vi "Application Analyzer.vi"() -> ()   [LabVIEW 2019]
doc: "Analyzes progress and status of application."
uses:
  <vilib>/Utility/error.llb/DialogType.ctl
  <vilib>/Utility/miscctls.llb/LVPointTypeDef.ctl
panel:
  out "Control Tab":T1(tab)
  out "Files & Revision":string[][](array[string])
  out "Total Revisions":u32
  out "Error Message":string
  out "Error Out":errorcluster
  out "VI-filename":string
  out "VI Path":path
  out "Revision Number":u32
  in  "Tool Bar:Visible":bool
  in  "Tabs Visible?":bool
  out "VI-Name":string
  # "Settings"
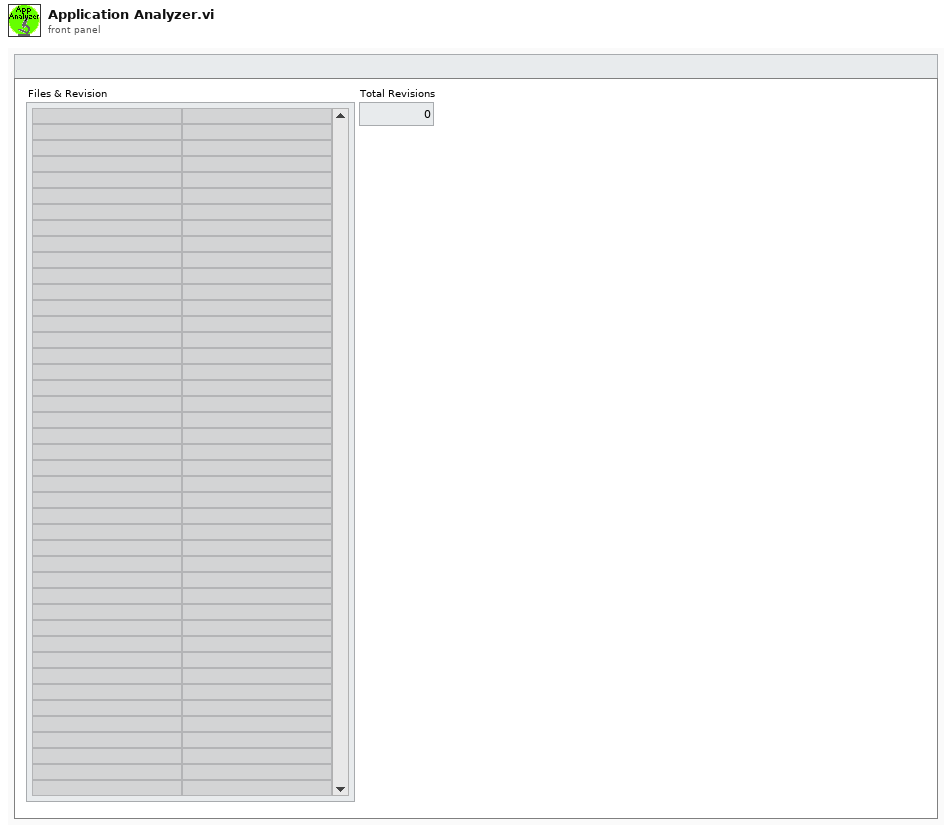
[diagram p1: front panel]
types:
  T1 = enum32{"GUI", "Controls & Indicators", "Error IO", "VI"}
  T2 = typedef "LVPointTypeDef.ctl" = cluster{"Horizontal":i16, "Vertical":i16}
  T3 = typedef "DialogType.ctl" = u16
  T4 = typedef "LVRectTypeDef.ctl" = cluster{"Left":i16, "Top":i16, "Right":i16, "Bottom":i16}
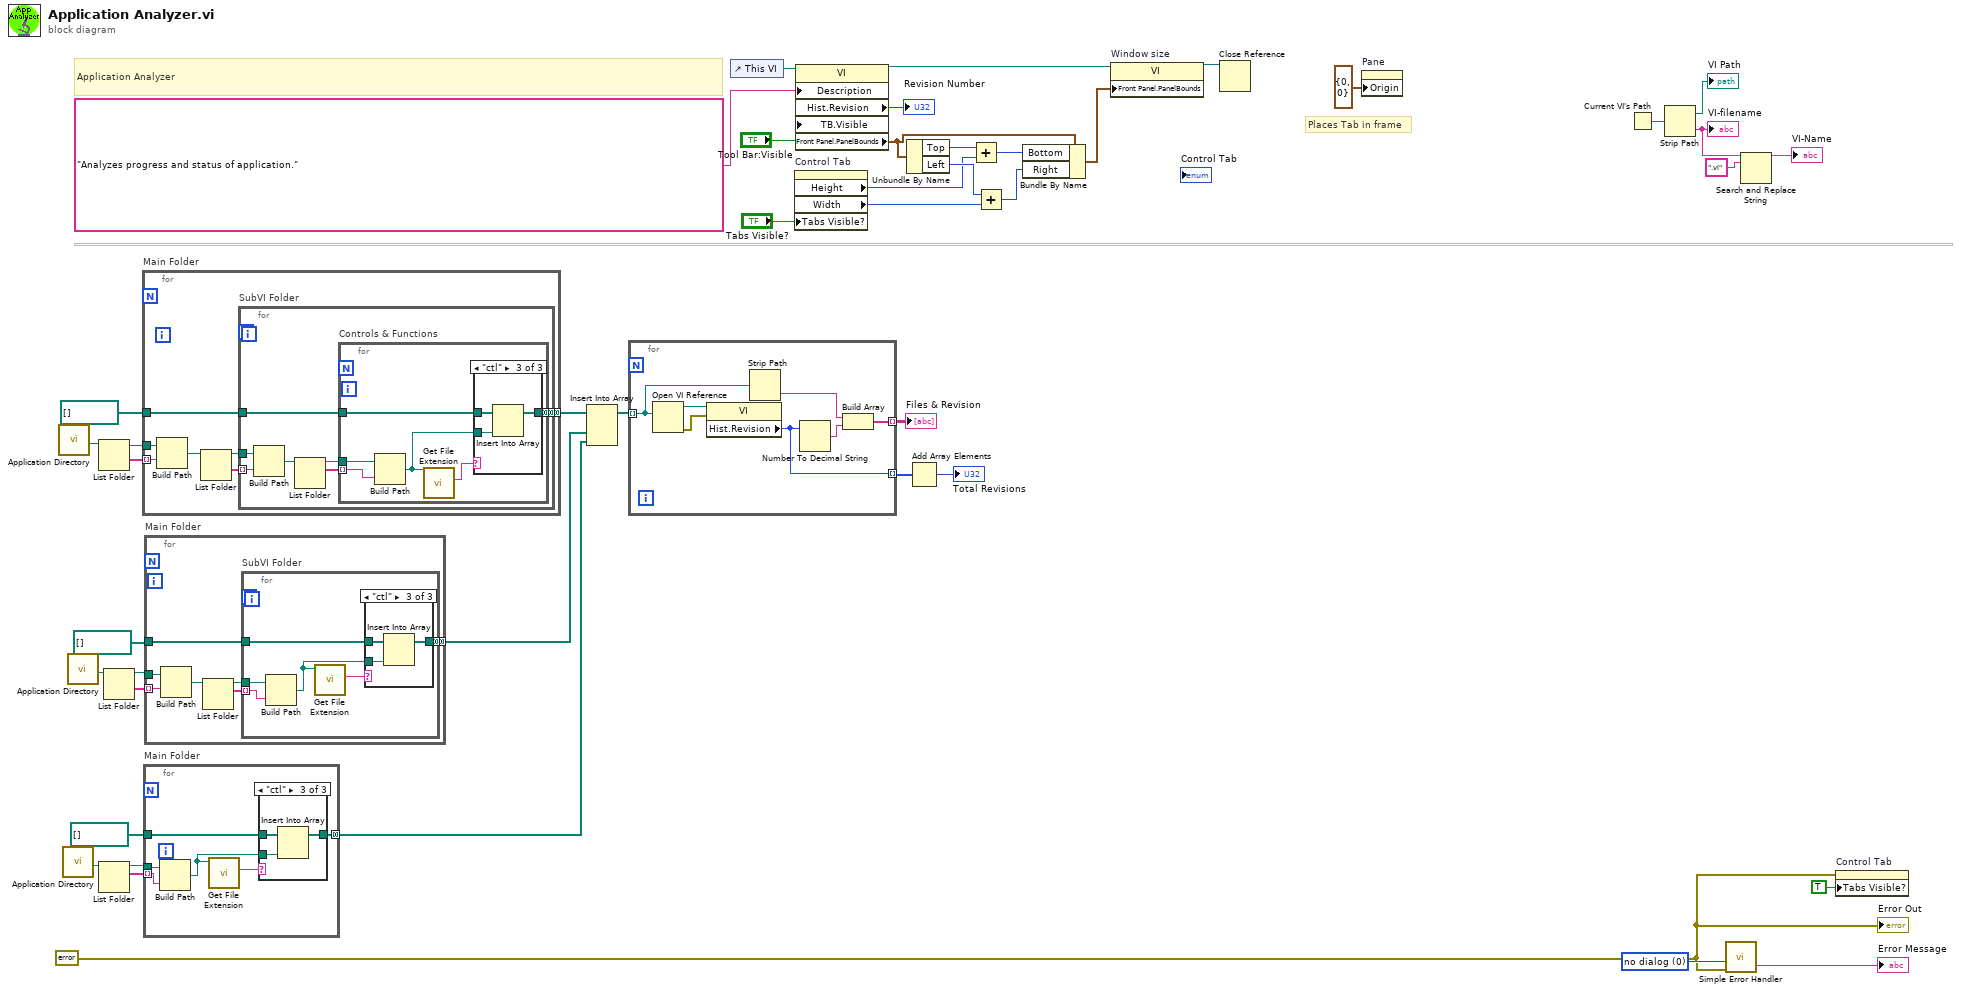
[diagram p0: block diagram]
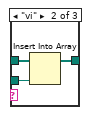
[diagram p3: hidden frame]
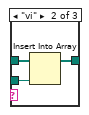
[diagram p5: hidden frame]
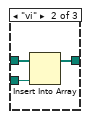
[diagram p7: hidden frame]
diagram:
  w32 = errorcluster {"status"=FALSE, "code"=0, "source"=""} ("Error In")
  w35 = T3 0 items=["no dialog", "OK message", "continue or stop message", "OK message + warnings", "continue/stop + warnings"] ("type of dialog (OK msg:1)")
  # "Places Tab in frame"
  # "Application Analyzer"
  n1 = call <vilib>:"Application Directory.vi"() -> ("Application Directory"=w17:path)
  n2 = call <vilib>:"Application Directory.vi"() -> ("Application Directory"=w12:path)
  n3 = call <vilib>:"Application Directory.vi"() -> ("Application Directory"=w16:path)
  n4 = List Folder(path=w17) -> (path out=w18:path, folder names=w19:string[])  [unwired: 3 in, 2 out]
  n5 = List Folder(path=w12) -> (path out=w13:path, filenames=w11:string[])  [unwired: 3 in, 2 out]
  n6 = List Folder(path=w16) -> (path out=w15:path, folder names=w14:string[])  [unwired: 3 in, 2 out]
  n7 = for "Main Folder" {
    tunnel: w19 -> [w51] mode=indexing
    tunnel: w18 -> [w46]
    tunnel: path[] [] -> [w47]
    tunnel: [w45] -> w6 mode=concatenating
    n8 = Build Path(base path=w46, name or relative path=w51) -> (appended path=w50:path)
    n9 = List Folder(path=w50) -> (path out=w48:path, folder names=w49:string[])  [unwired: 3 in, 2 out]
    n10 = for "SubVI Folder" {
      tunnel: w49 -> [w57] mode=indexing
      tunnel: w48 -> [w54]
      tunnel: w47 -> [w53]
      tunnel: [w52] -> w45 mode=concatenating
      n11 = Build Path(base path=w54, name or relative path=w57) -> (appended path=w58:path)
      n12 = List Folder(path=w58) -> (path out=w55:path, filenames=w56:string[])  [unwired: 3 in, 2 out]
      n13 = for "Controls & Functions" {
        tunnel: w56 -> [w62] mode=indexing
        tunnel: w55 -> [w64]
        tunnel: w53 -> [w61]
        tunnel: [w59] -> w52 mode=concatenating
        n14 = Build Path(base path=w64, name or relative path=w62) -> (appended path=w60:path)
        n15 = call <vilib>:"Get File Extension.vi"("file"=w60) -> ("lowercase file extension"=w63:string)  [unwired: 6 in, 4 out]
        n16 = case shown="\"ctl\"" w63 {
          tunnel: w61 -> [w65 w68 w71]
          tunnel: w60 -> [_ w66 w70]
          tunnel: [w65 w67 w69] -> w59
          frame "Other", Default {
          }
          frame "vi" {
            n17 = Insert Into Array(array=w68, new element=w66) -> (w67:path[])  [unwired: 1 in]
          }
          frame "ctl" {
            n18 = Insert Into Array(array=w71, new element=w70) -> (w69:path[])  [unwired: 1 in]
          }
        }
      }
    }
  }
  n19 = for "Main Folder" {
    tunnel: w13 -> [w73]
    tunnel: path[] [] -> [w77]
    tunnel: [w76] -> w4 mode=concatenating
    tunnel: w11 -> [w72] mode=indexing
    n20 = Build Path(base path=w73, name or relative path=w72) -> (appended path=w74:path)
    n21 = call <vilib>:"Get File Extension.vi"("file"=w74) -> ("lowercase file extension"=w75:string)  [unwired: 6 in, 4 out]
    n22 = case shown="\"ctl\"" w75 {
      tunnel: w77 -> [w78 w81 w84]
      tunnel: w74 -> [_ w79 w83]
      tunnel: [w78 w80 w82] -> w76
      frame "Other", Default {
      }
      frame "vi" {
        n23 = Insert Into Array(array=w81, new element=w79) -> (w80:path[])  [unwired: 1 in]
      }
      frame "ctl" {
        n24 = Insert Into Array(array=w84, new element=w83) -> (w82:path[])  [unwired: 1 in]
      }
    }
  }
  n25 = for "Main Folder" {
    tunnel: w14 -> [w91] mode=indexing
    tunnel: w15 -> [w86]
    tunnel: path[] [] -> [w87]
    tunnel: [w85] -> w5 mode=concatenating
    n26 = Build Path(base path=w86, name or relative path=w91) -> (appended path=w90:path)
    n27 = List Folder(path=w90) -> (path out=w89:path, filenames=w88:string[])  [unwired: 3 in, 2 out]
    n28 = for "SubVI Folder" {
      tunnel: w89 -> [w93]
      tunnel: w88 -> [w92] mode=indexing
      tunnel: w87 -> [w97]
      tunnel: [w96] -> w85 mode=concatenating
      n29 = Build Path(base path=w93, name or relative path=w92) -> (appended path=w94:path)
      n30 = call <vilib>:"Get File Extension.vi"("file"=w94) -> ("lowercase file extension"=w95:string)  [unwired: 6 in, 4 out]
      n31 = case shown="\"ctl\"" w95 {
        tunnel: w97 -> [w98 w101 w104]
        tunnel: w94 -> [_ w99 w103]
        tunnel: [w98 w100 w102] -> w96
        frame "Other", Default {
        }
        frame "vi" {
          n32 = Insert Into Array(array=w101, new element=w99) -> (w100:path[])  [unwired: 1 in]
        }
        frame "ctl" {
          n33 = Insert Into Array(array=w104, new element=w103) -> (w102:path[])  [unwired: 1 in]
        }
      }
    }
  }
  n34 = Insert Into Array(array=w6, new element #1=w5, new element #2=w4) -> (w3:path[])  [unwired: 1 in]
  n35 = for {
    tunnel: w3 -> [w111] mode=indexing
    tunnel: [w106] -> w2 mode=indexing
    tunnel: [w105] -> w10 mode=indexing
    n36 = Open VI Reference(vi path=w111) -> (vi reference=w109:refnum<vi>, error out=w110:errorcluster)  [unwired: 5 in]
    n37 = property class="VI"(reference=w109, error in=w110) -> ("Hist.Revision"=w106:u32)  [unwired: 2 out]
    n38 = Strip Path(path=w111) -> (name=w108:string)  [unwired: 1 out]
    n39 = Number To Decimal String(number=w106) -> (decimal integer string=w107:string)  [unwired: 1 in]
    n40 = Build Array(w108, w107) -> (w105:string[])
  }
  "Files & Revision" <- w10
  n41 = control-ref of="This VI"() -> (w41:refnum<vi>)
  n42 = property on="Control Tab" class="TabCtl (strict)"("Tabs Visible?"="Tabs Visible?") -> ("Height"=w26:u32, "Width"=w30:u32)  [unwired: 2 in, 2 out]
  n43 = property class="VI"(reference=w41, "Description"="Analyzes progress and status of application.", "TB.Visible"="Tool Bar:Visible") -> (reference out=w23:refnum<vi>, "Hist.Revision"=→"Revision Number":u32, "Front Panel.PanelBounds"=w24:T4)  [unwired: 1 in, 1 out]
  n44 = Unbundle By Name(w24) -> ("Top"=w25:i16, "Left"=w29:i16)
  n45 = Add Array Elements(numeric array=w2) -> (sum=→"Total Revisions":u32)
  n46 = Add(x=w25, y=w26) -> (x+y=w27:u32)
  n47 = Add(x=w29, y=w30) -> (x+y=w28:u32)
  n48 = Bundle By Name(cluster=w24, "Bottom"=w27, "Right"=w28) -> (w22:T4)
  n49 = property on="Window size" class="VI"(reference=w23, "Front Panel.PanelBounds"=w22) -> (reference out=w31:refnum<vi>)  [unwired: 1 in, 1 out]
  n50 = Close Reference(reference=w31) -> ()  [unwired: 1 in, 1 out]
  n51 = property on="Pane" class="Pane"("Origin"=T2 {"Horizontal"=0, "Vertical"=0}) -> ()  [unwired: 2 in, 2 out]
  n52 = Current VI's Path() -> (path=w44:path)
  n53 = Strip Path(path=w44) -> (stripped path=→"VI Path":path, name=w38:string)
  "VI-filename" <- w38
  n54 = call <vilib>:"Simple Error Handler.vi"("type of dialog (OK msg:1)"=w35, "error in (no error)"=w32) -> ("message"=→"Error Message":string)  [unwired: 3 in, 4 out]
  n55 = Search and Replace String(input string=w38, search string=".vi") -> (result string=→"VI-Name":string)  [unwired: 6 in, 3 out]
  n56 = property on="Control Tab" class="TabCtl (strict)"(error in=w32, "Tabs Visible?"=TRUE) -> ()  [unwired: 1 in, 2 out]
  "Error Out" <- w32
